vi "Set Axis Speed.vi"(9 "Speed (mm/s)":dbl=1.0, 10 "Axis":T1, 11 "VISA resource name":refnum<visa-resource-name>) -> ()   [LabVIEW 2011]
uses:
  Public/Utility/Axis Name.ctl
  Public/Utility/Serial Response Syntax.ctl
  ASI TG-1000.lvlib
panel:
  out "Command":string
  out "Command Accepted?":bool
  out "Response":string
  out "error out":errorcluster
  # "NB: this VI opens and closes the comm port"
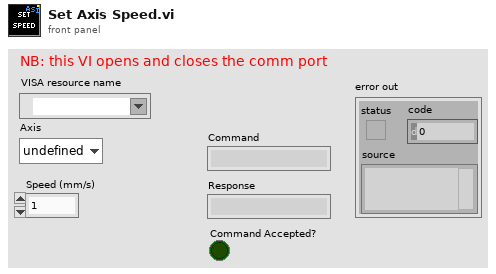
[diagram p1: front panel]
types:
  T1 = typedef "ASI TG-1000.lvlib/Axis Name.ctl" = enum8{"undefined", "A", "B", "C", "D", "E", "F", "G", "H", "I", "J", "K", "L", "M", "N", "O", "P", "Q", "R", "S", "T", "U", "V", "W", "X", "Y", "Z"}
  T2 = typedef "ASI TG-1000.lvlib/Serial Response Syntax.ctl" = enum16{":A then single line", "Single line, no :A", ":A or : then single line", ":A then single number", ":A or : then single number", ":A then <axis>= single number"}
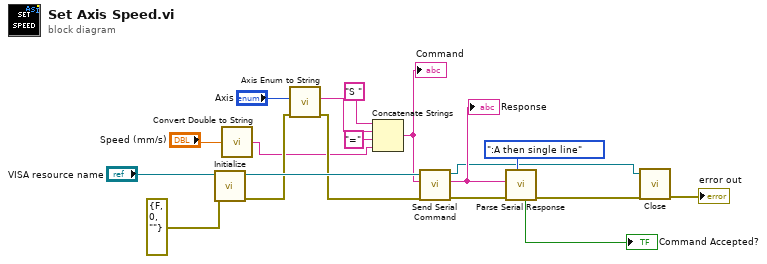
[diagram p0: block diagram]
diagram:
  n1 = call "Initialize.vi"("error in (no error)"=errorcluster {"status"=FALSE, "code"=0, "source"=""}, "VISA resource name"="VISA resource name") -> ("error out"=w13:errorcluster, "VISA resource name out"=w19:refnum<visa-resource-name>)  [unwired: 8 in]
  n2 = call "Convert Double to String.vi"("Value"="Speed (mm/s)") -> ("String"=w2:string)
  n3 = call "Axis Enum to String.vi"("error in (no error)"=w13, "Axis Enum In"="Axis") -> ("error out"=w12:errorcluster, "Axis String Out"=w11:string)  [unwired: 8 in]
  n4 = Concatenate Strings("S " ("Command"), w11, "=" ("string"), w2) -> (w9:string)
  "Command" <- w9
  n5 = call "Send Serial Command.vi"("error in (no error)"=w12, "Command"=w9, "VISA in"=w19) -> ("error out"=w7:errorcluster, "Response"=w5:string, "VISA out"=w4:refnum<visa-resource-name>)  [unwired: 6 in]
  "Response" <- w5
  n6 = call "Parse Serial Response.vi"("Response Syntax"=Serial_Response_Syntax.":A then single line", "error in (no error)"=w7, "Raw Response"=w5) -> ("error out"=w6:errorcluster, "As expected?"=→"Command Accepted?":bool)  [unwired: 5 in, 2 out]
  n7 = call "Close.vi"("error in (no error)"=w6, "VISA resource name"=w4) -> ("error out"=→"error out":errorcluster)  [unwired: 9 in]
